vi "PNS Variabler Taktmerker.vi"(8 "error in (no error)":errorcluster caption="Fehler (Eingang, kein Fehler)", 9 "Aus in sec.":dbl, 10 "Ein in sec.":dbl, 11 "Aktion":T1=enum."Lesen") -> (0 "error out":errorcluster caption="Fehler (Ausgang)", 2 "Takt":bool, 3 "Aktion":T1=enum."Lesen")   [LabVIEW 2015, in "PNS.lvlib"]
uses:
  PNS.lvlib
  Aktion PNS FGV variabler Taktmerker.ctl
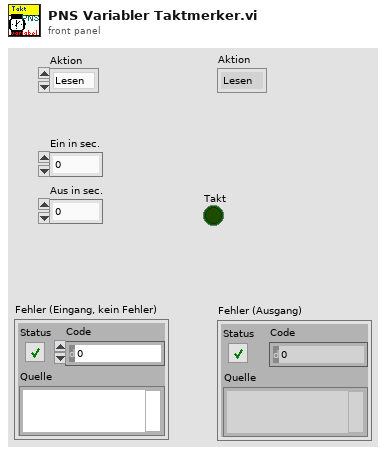
[diagram p1: front panel]
types:
  T1 = typedef "PNS.lvlib/Aktion PNS FGV variabler Taktmerker.ctl" = enum16{"Initialisieren", "Lesen", "aktiv", "inaktiv", "Werte schreiben"}
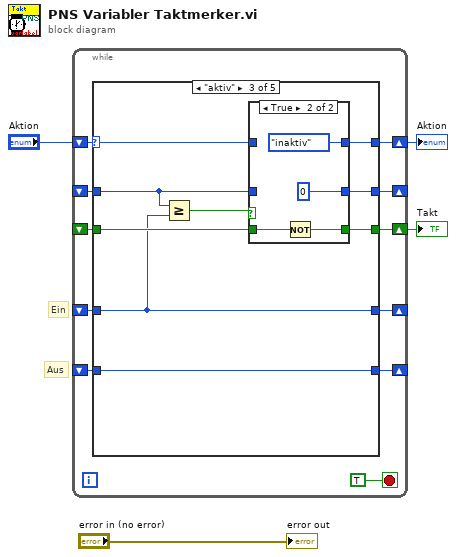
[diagram p0: block diagram]
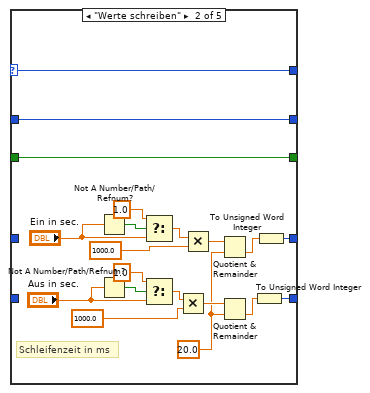
[diagram p3: hidden frame]
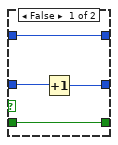
[diagram p4: hidden frame]
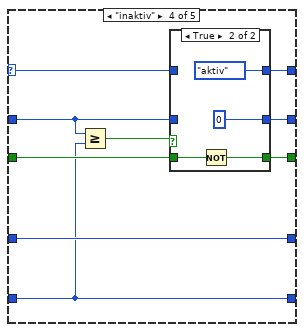
[diagram p5: hidden frame]
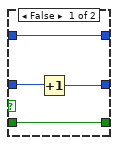
[diagram p6: hidden frame]
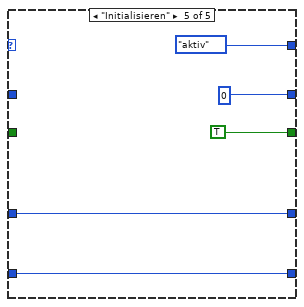
[diagram p7: hidden frame]
diagram:
  # "Aus"
  # "Ein"
  n1 = while {
    shift-right: [w13] -> _
    shift-left: _ -> [w12]
    shift-right: [w11] -> w2
    shift-left: _ -> [w10]
    shift-right: [w9] -> w3
    shift-left: "Aktion" -> [w14]
    shift-right: [w8] -> _
    shift-left: _ -> [w5]
    shift-right: [w7] -> _
    shift-left: _ -> [w6]
    stop <- TRUE stop-if-true
    n2 = case shown="\"aktiv\"" w14 {
      selector: w14 -> [w20 w40 w44 w61 _]
      tunnel: [w19 w39 w48 w65 u16 0 ("x+1")] -> w13
      tunnel: w12 -> [w19 w39 w47 w64 _]
      tunnel: [w18 w38 w46 w63 TRUE] -> w11
      tunnel: w10 -> [w18 w38 w45 w62 _]
      tunnel: [w20 w40 w43 w60 Aktion_PNS_FGV_variabler_Taktmerker."aktiv" ("Aktion")] -> w9
      tunnel: [w17 w30 w41 w59 w76] -> w8
      tunnel: [w16 w29 w42 w58 w75] -> w7
      tunnel: w6 -> [w16 _ w42 w58 w75]
      tunnel: w5 -> [w17 _ w41 w59 w76]
      frame "Lesen", Default {
      }
      frame "Werte schreiben" {
        w32 = 20.0 ("y")
        # "Schleifenzeit in ms"
        n3 = Not A Number/Path/Refnum?(number/path/refnum="Ein in sec.") -> (NaN/Path/Refnum?=w28:bool)
        n4 = Not A Number/Path/Refnum?(number/path/refnum="Aus in sec.") -> (NaN/Path/Refnum?=w23:bool)
        n5 = Select(t=1.0, s=w28, f="Ein in sec.") -> (s? t:f=w25:dbl)
        n6 = Select(t=1.0, s=w23, f="Aus in sec.") -> (s? t:f=w22:dbl)
        n7 = Multiply(x=w22, y=1000.0) -> (x*y=w34:dbl)
        n8 = Multiply(x=w25, y=1000.0) -> (x*y=w35:dbl)
        n9 = Quotient & Remainder(x=w35, y=w32) -> (floor(x/y)=w33:dbl)  [unwired: 1 out]
        n10 = Quotient & Remainder(x=w34, y=w32) -> (floor(x/y)=w31:dbl)  [unwired: 1 out]
        n11 = To Unsigned Word Integer(number=w31) -> (unsigned 16bit integer=w29:u16)
        n12 = To Unsigned Word Integer(number=w33) -> (unsigned 16bit integer=w30:u16)
      }
      frame "aktiv" {
        n13 = Greater Or Equal?(x=w47, y=w41) -> (x >= y?=w49:bool)
        n14 = case shown="True" w49 {
          tunnel: [w52 u16 0 ("x+1")] -> w48
          tunnel: w47 -> [w53 _]
          tunnel: [w51 w56] -> w46
          tunnel: w45 -> [w51 w55]
          tunnel: w44 -> [w50 _]
          tunnel: [w50 Aktion_PNS_FGV_variabler_Taktmerker."inaktiv" ("Aktion")] -> w43
          frame False {
            n15 = Increment(x=w53) -> (x+1=w52:u16)
          }
          frame True {
            n16 = Not(x=w55) -> (.not. x?=w56:bool)
          }
        }
      }
      frame "inaktiv" {
        n17 = Greater Or Equal?(x=w64, y=w58) -> (x >= y?=w66:bool)
        n18 = case shown="True" w66 {
          tunnel: [w69 u16 0 ("x+1")] -> w65
          tunnel: w64 -> [w70 _]
          tunnel: [w68 w73] -> w63
          tunnel: w62 -> [w68 w72]
          tunnel: w61 -> [w67 _]
          tunnel: [w67 Aktion_PNS_FGV_variabler_Taktmerker."aktiv" ("Aktion")] -> w60
          frame False {
            n19 = Increment(x=w70) -> (x+1=w69:u16)
          }
          frame True {
            n20 = Not(x=w72) -> (.not. x?=w73:bool)
          }
        }
      }
      frame "Initialisieren" {
      }
    }
  }
  "Aktion" <- w3
  "Takt" <- w2
  "error out" <- "error in (no error)"
